vi "Get_N_Steps.vi"(2 "Increment":dbl, 3 "Lower Limit":dbl, 4 "Upper Limit":dbl) -> (0 "Bounds Are Good":bool, 1 "N steps":i32)   [LabVIEW 2019]
doc: "Given a set [xl, xu] and you want to use dx, how many steps are required? \n\nR. Sheehan 21 - 4 - 2015"
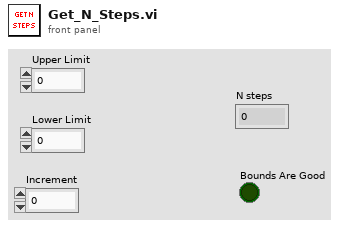
[diagram p1: front panel]
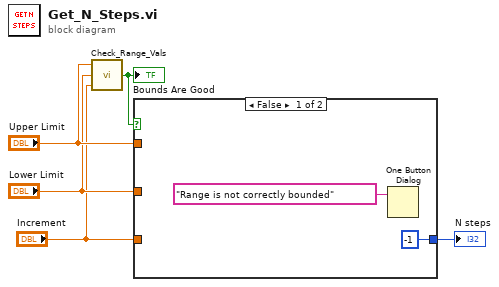
[diagram p0: block diagram]
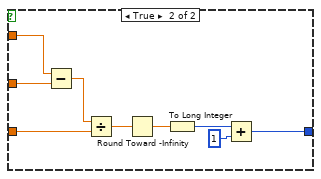
[diagram p2: hidden frame]
diagram:
  n1 = call "Check_Range_Vals.vi"("Increment"="Increment", "Lower Limit"="Lower Limit", "Upper Limit"="Upper Limit") -> ("Bounds Are Good"=w5:bool)
  "Bounds Are Good" <- w5
  n2 = case shown="False" w5 {
    tunnel: "Upper Limit" -> [_ w16]
    tunnel: "Lower Limit" -> [_ w15]
    tunnel: "Increment" -> [_ w13]
    tunnel: [-1 w8] -> w1
    frame False {
      n3 = One Button Dialog(message="Range is not correctly bounded") -> ()  [unwired: 1 in, 1 out]
    }
    frame True {
      n4 = Subtract(x=w16, y=w15) -> (x-y=w14:dbl)
      n5 = Divide(x=w14, y=w13) -> (x/y=w12:dbl)
      n6 = Round Toward -Infinity(1:w12) -> (0:w11:dbl)
      n7 = To Long Integer(number=w11) -> (32bit integer=w9:i32)
      n8 = Add(x=w9, y=1) -> (x+y=w8:i32)
    }
  }
  "N steps" <- w1
